vi "NT to XML Number.vi"(10 "NT Name":string="Magazine_Firing_Power", 11 "XML File Path":path=path "/home/lvuser/natinst/bin/Cals/Drive.XML") -> (2 "Numeric":dbl)   [LabVIEW 2020]
uses:
  <vilib>/Rock Robotics/Network Tables/NT Read Number.vi
  <vilib>/Utility/xml.llb/Write to XML File(string).vi
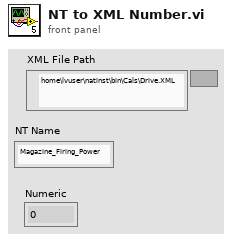
[diagram p1: front panel]
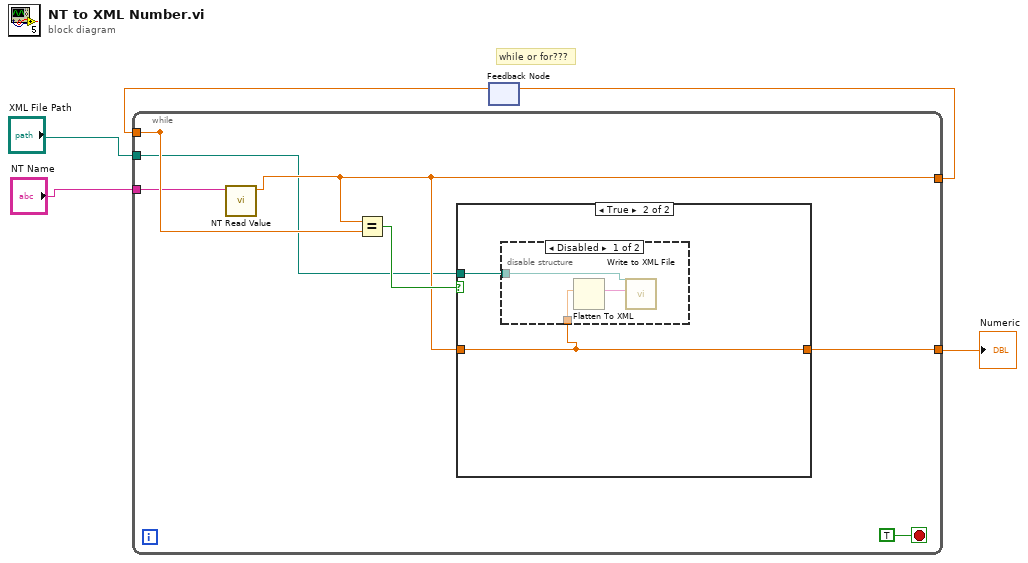
[diagram p0: block diagram]
diagram:
  # "while or for???"
  n1 = feedback #1() -> (w4:dbl)  [unwired: 1 in]
  n2 = while {
    tunnel: [w7] -> w5
    tunnel: [w12] -> _
    tunnel: w4 -> [w12]
    tunnel: "NT Name" -> [w9]
    tunnel: [w8] -> w2
    tunnel: "XML File Path" -> [w6]
    stop <- TRUE stop-if-true
    n3 = call-poly <vilib>:"NT Read Value.vi"("Name"=w9) -> ("Numeric"=w7:dbl)  [unwired: 9 in, 1 out]
    n4 = Equal?(x=w7, y=w12) -> (x = y?=w11:bool)
    n5 = case shown="True" w11 {
      tunnel: [w13 w15] -> w8
      tunnel: w7 -> [w13 w15]
      tunnel: w6 -> [_ w14]
      frame False {
      }
      frame True {
        n6 = disable-structure shown="Disabled" {
          disable-tunnel: w15 -> [w18 _]
          disable-tunnel: w14 -> [w16 _]
          frame Disabled {
            n7 = Flatten To XML(anything=w18) -> (xml string=w17:string)
            n8 = call-poly <vilib>:"Write to XML File.vi"("XML Input"=w17, "XML File Path"=w16) -> ()  [unwired: 7 in, 3 out]
          }
          frame Enabled {
          }
        }
      }
    }
  }
  "Numeric" <- w2
  n9 = feedback-in #1(w5) -> ()
